vi "EverythingMultiFPGATest.vi"() -> ()   [LabVIEW 2017]
uses:
  Version Token.ctl
  Analog Replay/Settings.ctl
  Analog Replay/Input.ctl
  Analog Replay/Load Input.ctl
  Digital Pattern Generation/Load Input.ctl
  Digital Pattern Generation/Settings.ctl
  Digital Pattern Generation/Input.ctl
  ECU Event/Timing/Measure Output.ctl
  ECU Event/Timing/Measure Settings.ctl
  ECU Event/Timing/Capture Output.ctl
  Knock Sensor/Generate Input.ctl
  Knock Sensor/Cylinder Input.ctl
  Knock Sensor/Cylinder Settings.ctl
  Knock Sensor/Generate Settings.ctl
  Directional Speed/Load Input.ctl
  Directional Speed/Settings.ctl
  Directional Speed/Input.ctl
  APU/Settings.ctl
  APU/Input.ctl
  APU/Output.ctl
  APU/Shared Settings.ctl
  <vilib>/Platform/TimedLoop/XDataNode/timing_clust.ctl
  <vilib>/Platform/TimedLoop/XDataNode/nitl_modes.ctl
  <vilib>/Platform/TimedLoop/XDataNode/wakeup.ctl
  ECU Event/Timing/Capture Settings.ctl
  <vilib>/rvi/Emulation/niFpgaGetClockAttributes.vi
  <vilib>/rvi/Emulation/niFpgaSctlEmulationGetInTimedLoop.vi
  <vilib>/rvi/Emulation/niFpgaEmulationReportErrorSimple.vi
  <vilib>/rvi/DataTransferAndStorage/Container/Common/niFpgaContainerGetUniqueNameForEmu.vi
  <vilib>/rvi/DataTransferAndStorage/Container/Common/niFpgaContainerSetEmuInfo.vi
  <vilib>/rvi/eio/common/nirviEmuReportErrorAndStop.vi
  <vilib>/rvi/Emulation/niFpgaCriticalErrorInLSC.vi
  <vilib>/rvi/eio/common/nirviEmuTemplateMethod_errors.vi
  ECU Event/Timing/Measure Events (40MHz).vi
  <vilib>/rvi/DataTransferAndStorage/Container/Common/niFpgaContainerExecOnDevCompGetState.vi
  <vilib>/rvi/Emulation/niFpgaEmulationIsFPGAContextNoSignature.vi
  <vilib>/rvi/Memory/Memory_Emulation/niFpgaMemoryEmulationCacheClearOnFirstRun.vi
  <vilib>/rvi/Memory/Memory_Emulation/nirvimemoryEmulationManagerCache_MakeExclusive.vi
  <vilib>/rvi/Memory/Memory_Emulation/niFpgaMemoryEmulationValidateCache.vi
  <vilib>/rvi/Memory/Memory_Emulation/nirvimemoryEmulationManagerCache_InsertValue.vi
  <vilib>/Utility/error.llb/Clear Errors.vi
  <vilib>/rvi/Memory/Memory_Emulation/nirvimemoryEmulationManagerCache_ReleaseExclusive.vi
  <vilib>/rvi/Memory/Memory_Emulation/nirvimemoryEmulationManagerCache_GetValue.vi
  <vilib>/rvi/Memory/Memory_Emulation/nirvimemoryEmulationManagerCache_SetValue.vi
  <vilib>/rvi/Emulation/niFpgaProcessEmulError.vi
  <vilib>/rvi/LocalResourceManager/LocalResourceManager.xnode
  <vilib>/Platform/TimedLoop/XDataNode/XDataNode.xnode
  <vilib>/eio/EIONode/EIONode.xnode
  <vilib>/rvi/DataTransferAndStorage/Container/XNode/niFpgaContainer.xnode
  <vilib>/rvi/DataTransferAndStorage/Register/Emulation/niFpgaRegisterEmulationRefIn.vi
  <vilib>/Platform/TimedLoop/XDataNode/XDNodeRunTimeDep.lvlib
  Analog Replay/Analog Replay.lvlib
  Digital Pattern Generation/Digital Pattern Generation.lvlib
  ECU Event/Timing/ECU Event Timing.lvlib
  Knock Sensor/Knock Sensor.lvlib
  Directional Speed/Directional Speed.lvlib
  APU/APU.lvlib
  Engine Simulation Toolkit.lvlib
panel:
  in  "trigger line.apu 1":refnum<k21>="PXI_Trig0"
  in  "send trigger.apu 1":bool
  in  "shared settings.apu 1":T1 {"start" format="%#.15g"}
  in  "go.apu 1":bool
  in  "master.apu 1":bool
  out "output.apu 1":T2 caption="output"
  in  "input.apu 1":T3={"desired speed"=0.0, "reset"=TRUE} caption="input"
  in  "settings.apu 1":T4 caption="settings"
  out "Digital Pattern Test.apu 1":T5
  in  "load input.Dir Speed DIO0":T6
  in  "input.Dir Speed DIO0":T7
  in  "settings.Dir Speed DIO0":T8
  in  "input.Dir Speed DIO1":T7
  in  "settings.Dir Speed DIO1":T8
  in  "load input.Dir Speed DIO1":T6
  in  "settings.Knock AO 3":T9
  in  "settings.Knock AO 3.Cylinder 1":T10
  in  "settings.Knock AO 3.Cylinder 2":T10
  in  "settings.Knock AO 3.Cylinder 3":T10
  in  "settings.Knock AO 3.Cylinder 4":T10
  in  "input.Knock AO 3.Cylinder 1":T11
  in  "input.Knock AO 3.Cylinder 2":T11
  in  "input.Knock AO 3.Cylinder 3":T11
  in  "input.Knock AO 3.Cylinder 4":T11
  in  "input.Knock AO 3":T12
  in  "settings.Knock AO 3.Cylinder 5":T10
  in  "settings.Knock AO 3.Cylinder 6":T10
  in  "input.Knock AO 3.Cylinder 5":T11
  in  "input.Knock AO 3.Cylinder 6":T11
  in  "settings.Knock AO 2.Cylinder 5":T10
  in  "settings.Knock AO 2.Cylinder 6":T10
  in  "input.Knock AO 2.Cylinder 5":T11={"probability compare"=65535, "high freq scaler"=0.0, "trigger position"=0}
  in  "input.Knock AO 2.Cylinder 6":T11={"probability compare"=65535, "high freq scaler"=0.0, "trigger position"=0}
  in  "settings.Knock AO 2":T9
  in  "settings.Knock AO 2.Cylinder 1":T10
  in  "settings.Knock AO 2.Cylinder 2":T10
  in  "settings.Knock AO 2.Cylinder 3":T10
  in  "settings.Knock AO 2.Cylinder 4":T10
  in  "input.Knock AO 2.Cylinder 1":T11={"probability compare"=65535, "high freq scaler"=0.0, "trigger position"=0}
  in  "input.Knock AO 2.Cylinder 2":T11={"probability compare"=65535, "high freq scaler"=0.0, "trigger position"=0}
  in  "input.Knock AO 2.Cylinder 3":T11={"probability compare"=65535, "high freq scaler"=0.0, "trigger position"=0}
  in  "input.Knock AO 2.Cylinder 4":T11={"probability compare"=65535, "high freq scaler"=0.0, "trigger position"=0}
  in  "input.Knock AO 2":T12
  out "capture.Multi Event DIO 15.Event 4":T13
  out "capture.Multi Event DIO 15.Event 3":T13
  out "capture.Multi Event DIO 15.Event 2":T13
  out "capture.Multi Event DIO 14.Event 4":T13
  out "capture.Multi Event DIO 14.Event 3":T13
  out "capture.Multi Event DIO 14.Event 2":T13
  out "capture.Multi Event DIO 13.Event 4":T13
  out "capture.Multi Event DIO 13.Event 3":T13
  out "capture.Multi Event DIO 13.Event 2":T13
  out "capture.Multi Event DIO 12.Event 4":T13
  out "capture.Multi Event DIO 12.Event 3":T13
  out "capture.Multi Event DIO 12.Event 2":T13
  out "capture.Multi Event DIO 11.Event 4":T13
  out "capture.Multi Event DIO 11.Event 3":T13
  out "capture.Multi Event DIO 11.Event 2":T13
  out "capture.Multi Event DIO 10.Event 4":T13
  out "capture.Multi Event DIO 10.Event 3":T13
  out "capture.Multi Event DIO 10.Event 2":T13
  out "capture.Multi Event DIO 10.Event 1":T13
  out "capture.Multi Event DIO 11.Event 1":T13
  out "capture.Multi Event DIO 12.Event 1":T13
  out "capture.Multi Event DIO 13.Event 1":T13
  out "capture.Multi Event DIO 14.Event 1":T13
  out "capture.Multi Event DIO 15.Event 1":T13
  in  "settings.Multi Event DIO 10":T14
  in  "settings.Multi Event DIO 11":T14
  in  "settings.Multi Event DIO 12":T14
  in  "settings.Multi Event DIO 13":T14
  in  "settings.Multi Event DIO 14":T14
  in  "settings.Multi Event DIO 15":T14
  out "status.Multi Event DIO 10":T15
  out "status.Multi Event DIO 11":T15
  out "status.Multi Event DIO 12":T15
  out "status.Multi Event DIO 13":T15
  out "status.Multi Event DIO 14":T15
  out "status.Multi Event DIO 15":T15
  out "capture.Event DIO 4.Event 1":T13
  out "capture.Event DIO 5.Event 1":T13
  out "capture.Event DIO 6.Event 1":T13
  out "capture.Event DIO 7.Event 1":T13
  out "capture.Event DIO 8.Event 1":T13
  out "capture.Event DIO 9.Event 1":T13
  in  "settings.Event DIO 4":T14
  in  "settings.Event DIO 5":T14
  in  "settings.Event DIO 6":T14
  in  "settings.Event DIO 7":T14
  in  "settings.Event DIO 8":T14
  in  "settings.Event DIO 9":T14
  out "status.Event DIO 4":T15
  out "status.Event DIO 5":T15
  out "status.Event DIO 6":T15
  out "status.Event DIO 7":T15
  out "status.Event DIO 8":T15
  out "status.Event DIO 9":T15
  in  "load input.Pattern DIO 3":T16
  in  "load input.Pattern DIO 2":T16
  in  "load input.Pattern DIO 1":T16
  in  "input.Pattern DIO 0":T17
  in  "settings.Pattern DIO 0":T18
  in  "input.Pattern DIO 1":T17
  in  "settings.Pattern DIO 1":T18
  in  "input.Pattern DIO 2":T17
  in  "settings.Pattern DIO 2":T18
  in  "input.Pattern DIO 3":T17
  in  "settings.Pattern DIO 3":T18
  in  "load input.Pattern DIO 0":T16
  in  "load input.replay AO 1":T19={"Data"=[0, 0, 0, 0, 0, 0, 0, 0, 0, 0, 0, 0, 0, 0, 0, 0], "LoadOffset"=0, "Done"=FALSE} caption="input"
  in  "load input.replay AO 0":T19={"Data"=[0, 0, 0, 0, 0, 0, 0, 0, 0, 0, 0, 0, 0, 0, 0, 0], "LoadOffset"=0, "Done"=FALSE} caption="input"
  in  "input.replay AO 0":T20 caption="input"
  in  "input.replay AO 1":T20 caption="input"
  in  "settings.replay AO 1":T21 caption="settings"
  in  "settings.replay AO 0":T21 caption="settings"
  in  "est.version":T22
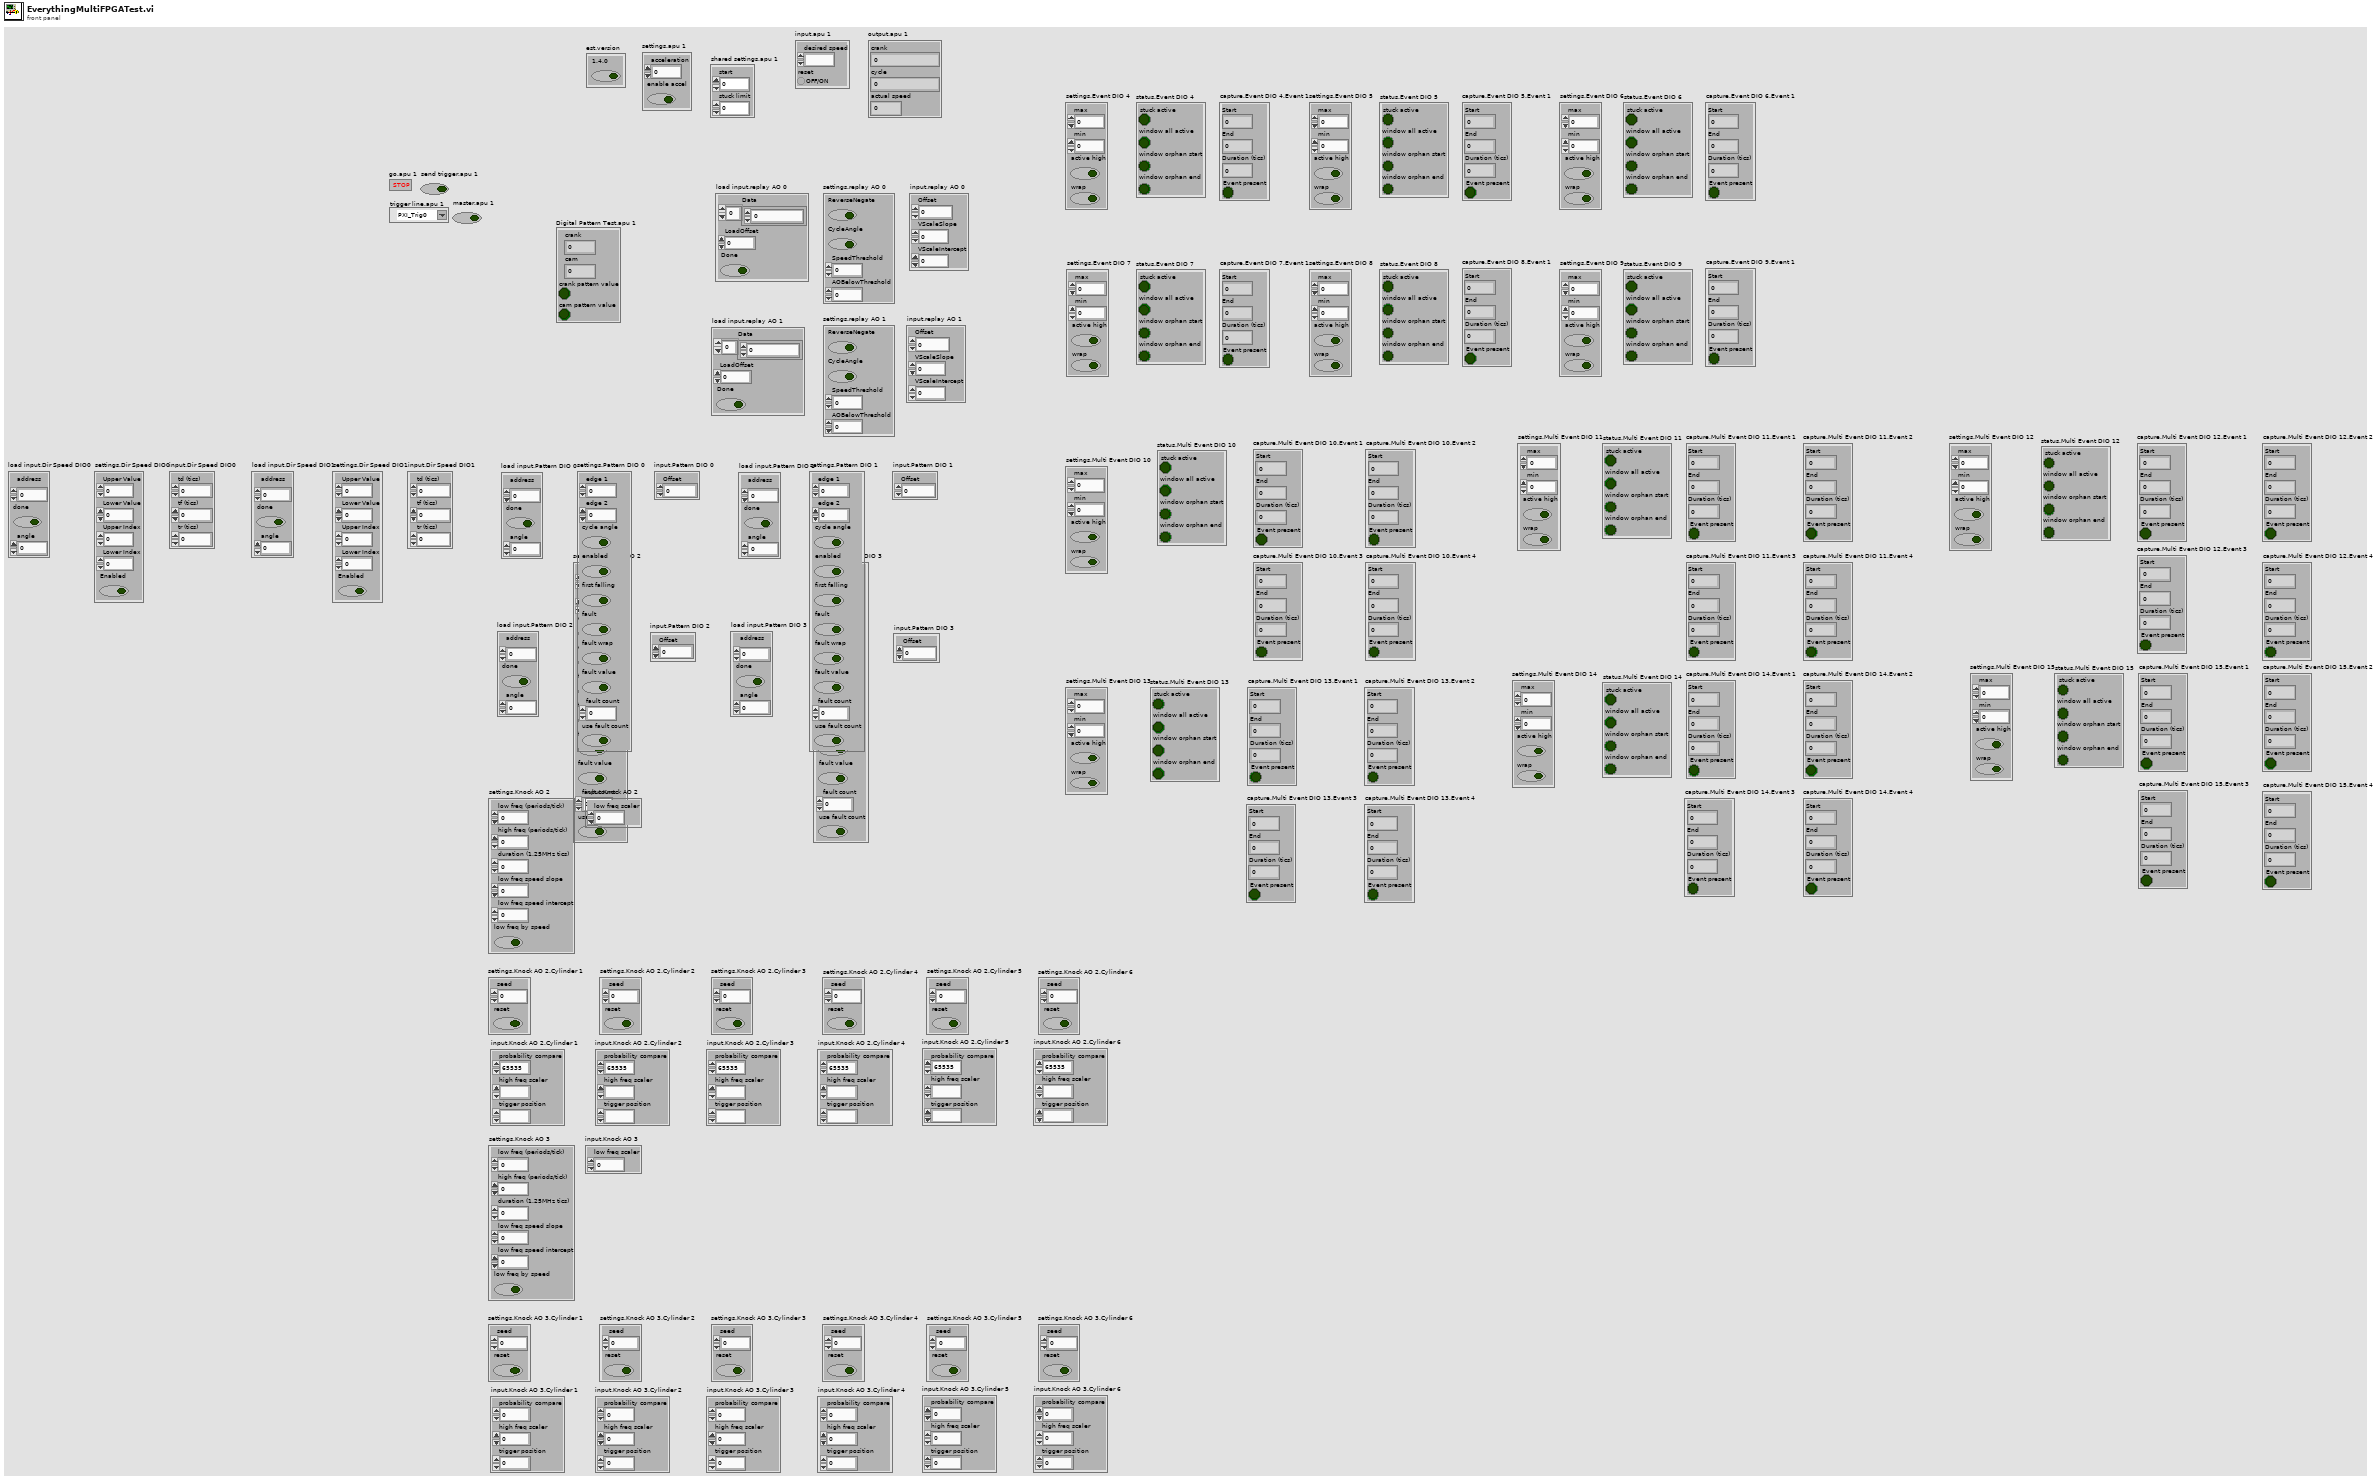
[diagram p1: front panel]
types:
  T1 = typedef "Engine Simulation Toolkit.lvlib/APU.lvlib/Shared Settings.ctl" = cluster{"start":fxp<+,17,17>, "stuck limit":fxp<+,18,18>}
  T2 = typedef "Engine Simulation Toolkit.lvlib/APU.lvlib/Output.ctl" = cluster{"crank":u16, "cycle":u16, "actual speed":fxp<+/-,23,2>}
  T3 = typedef "Engine Simulation Toolkit.lvlib/APU.lvlib/Input.ctl" = cluster{"desired speed":fxp<+/-,23,2>, "reset":bool}
  T4 = typedef "Engine Simulation Toolkit.lvlib/APU.lvlib/Settings.ctl" = cluster{"acceleration":fxp<+,18,-20>, "enable accel":bool}
  T5 = cluster{"crank":u16, "cam":u16, "crank pattern value":bool, "cam pattern value":bool}
  T6 = typedef "Engine Simulation Toolkit.lvlib/Directional Speed.lvlib/Load Input.ctl" = cluster{"address":fxp<+,10,10>, "done":bool, "angle":u16}
  T7 = typedef "Engine Simulation Toolkit.lvlib/Directional Speed.lvlib/Input.ctl" = cluster{"td (tics)":u16, "tf (tics)":u16, "tr (tics)":u16}
  T8 = typedef "Engine Simulation Toolkit.lvlib/Directional Speed.lvlib/Settings.ctl" = cluster{"Upper Value":u16, "Lower Value":u16, "Upper Index":fxp<+,10,10>, "Lower Index":fxp<+,10,10>, "Enabled":bool}
  T9 = typedef "Engine Simulation Toolkit.lvlib/Knock Sensor.lvlib/Generate Settings.ctl" = cluster{"low freq (periods/tick)":fxp<+,32,0>, "high freq (periods/tick)":fxp<+,32,0>, "duration (1.25MHz tics)":fxp<+,18,18>, "low freq speed slope":fxp<+,16,-3>, "low freq speed intercept":fxp<+,10,-10>, "low freq by speed":bool}
  T10 = typedef "Engine Simulation Toolkit.lvlib/Knock Sensor.lvlib/Cylinder Settings.ctl" = cluster{"seed":u16, "reset":bool}
  T11 = typedef "Engine Simulation Toolkit.lvlib/Knock Sensor.lvlib/Cylinder Input.ctl" = cluster{"probability compare":u16, "high freq scaler":fxp<+,10,0>, "trigger position":u16}
  T12 = typedef "Engine Simulation Toolkit.lvlib/Knock Sensor.lvlib/Generate Input.ctl" = cluster{"low freq scaler":fxp<+,10,0>}
  T13 = typedef "Engine Simulation Toolkit.lvlib/ECU Event Timing.lvlib/Capture Output.ctl" = cluster{"Start":u16, "End":u16, "Duration (tics)":fxp<+,18,18>, "Event present":bool}
  T14 = typedef "Engine Simulation Toolkit.lvlib/ECU Event Timing.lvlib/Measure Settings.ctl" = cluster{"max":u16, "min":u16, "active high":bool, "wrap":bool}
  T15 = typedef "Engine Simulation Toolkit.lvlib/ECU Event Timing.lvlib/Measure Output.ctl" = cluster{"stuck active":bool, "window all active":bool, "window orphan start":bool, "window orphan end":bool}
  T16 = typedef "Engine Simulation Toolkit.lvlib/Digital Pattern Generation.lvlib/Load Input.ctl" = cluster{"address":fxp<+,11,11>, "done":bool, "angle":u16}
  T17 = typedef "Engine Simulation Toolkit.lvlib/Digital Pattern Generation.lvlib/Input.ctl" = cluster{"Offset":i16}
  T18 = typedef "Engine Simulation Toolkit.lvlib/Digital Pattern Generation.lvlib/Settings.ctl" = cluster{"edge 1":u16, "edge 2":u16, "cycle angle":bool, "enabled":bool, "first falling":bool, "fault":bool, "fault wrap":bool, "fault value":bool, "fault count":fxp<+,4,4>, "use fault count":bool}
  T19 = typedef "Engine Simulation Toolkit.lvlib/Analog Replay.lvlib/Load Input.ctl" = cluster{"Data":i16[], "LoadOffset":u16, "Done":bool}
  T20 = typedef "Engine Simulation Toolkit.lvlib/Analog Replay.lvlib/Input.ctl" = cluster{"Offset":i16, "VScaleSlope":fxp<+,18,6>, "VScaleIntercept":fxp<+/-,18,3>}
  T21 = typedef "Engine Simulation Toolkit.lvlib/Analog Replay.lvlib/Settings.ctl" = cluster{"ReverseNegate":bool, "CycleAngle":bool, "SpeedThreshold":fxp<+/-,23,2>, "AOBelowThreshold":i16}
  T22 = typedef "Engine Simulation Toolkit.lvlib/Version Token.ctl" = cluster{"1.4.0":bool}
  T23 = typedef "XDNodeRunTimeDep.lvlib/timing_clust.ctl" = cluster{"Expected End [f-1]":u64, "Actual End [f-1]":u64, "Finished Late? [f-1]":bool, "Expected End [i-1]":u64, "Actual End [i-1]":u64, "Finished Late? [i-1]":bool, "Expected Start [i]":u64, "Actual Start [i]":u64, "Expected Start [f]":u64, "Actual Start [f]":u64, "Source Name":string, "Structure Name":string, "Period":i64, "Deadline":i64, "Offset":i64, "Start":i64, "Priority":i32, "Timeout":i32, "Mode":T24, "Wakeup Reason":T25, "Error":errorcluster, "Source Type":string, "Secondary Source Type":string, "Global End Time":u64, "Global Start Time":u64, "Frame Duration":u64, "Iteration Duration":u64, "Assigned CPU":i32, "I/O Scan Engine Mode":u32}
  T24 = typedef "XDNodeRunTimeDep.lvlib/nitl_modes.ctl" = enum32{"No Change", "Process missed periods, maintain original phase", "Discard missed periods, maintain original phase", "Process missed periods, ignore original phase", "Discard missed periods, ignore original phase"}
  T25 = typedef "XDNodeRunTimeDep.lvlib/wakeup.ctl" = enum32{"Normal", "Aborted", "Asynchronous wakeup", "Timing source error", "Timed loop error", "Timeout"}
  T26 = typedef "Engine Simulation Toolkit.lvlib/Directional Speed.lvlib/Load Data.ctl" = cluster{"max address":fxp<+,10,10>, "Memory":refnum<k21>}
  T27 = typedef "Engine Simulation Toolkit.lvlib/APU.lvlib/Register Bus.ctl" = cluster{"Speed":refnum<k21>, "Crank Angle":refnum<k21>, "Cycle Angle":refnum<k21>, "Crank Count":refnum<k21>, "Cycle Count":refnum<k21>, "1.25 MHz Counter":refnum<k21>, "Crank Rollover":refnum<k21>, "Cycle Rollover":refnum<k21>, "shared settings":T1}
  T28 = typedef "Engine Simulation Toolkit.lvlib/Digital Pattern Generation.lvlib/Load Data.ctl" = cluster{"max address":fxp<+,11,11>, "memory":refnum<k21>}
  T29 = typedef "Engine Simulation Toolkit.lvlib/Knock Sensor.lvlib/Triggered Cylinder Data.ctl" = cluster{"trigger knock":bool, "high freq scaler":fxp<+,10,0>}
  T30 = typedef "Engine Simulation Toolkit.lvlib/ECU Event Timing.lvlib/Capture Settings.ctl" = u8
  T31 = typedef "Engine Simulation Toolkit.lvlib/ECU Event Timing.lvlib/Measured Data.ctl" = cluster{"start":u16, "end":u16, "duration (tics)":fxp<+,18,18>, "window end":bool, "window begin":bool, "pulse end":bool, "pulse #":u8}
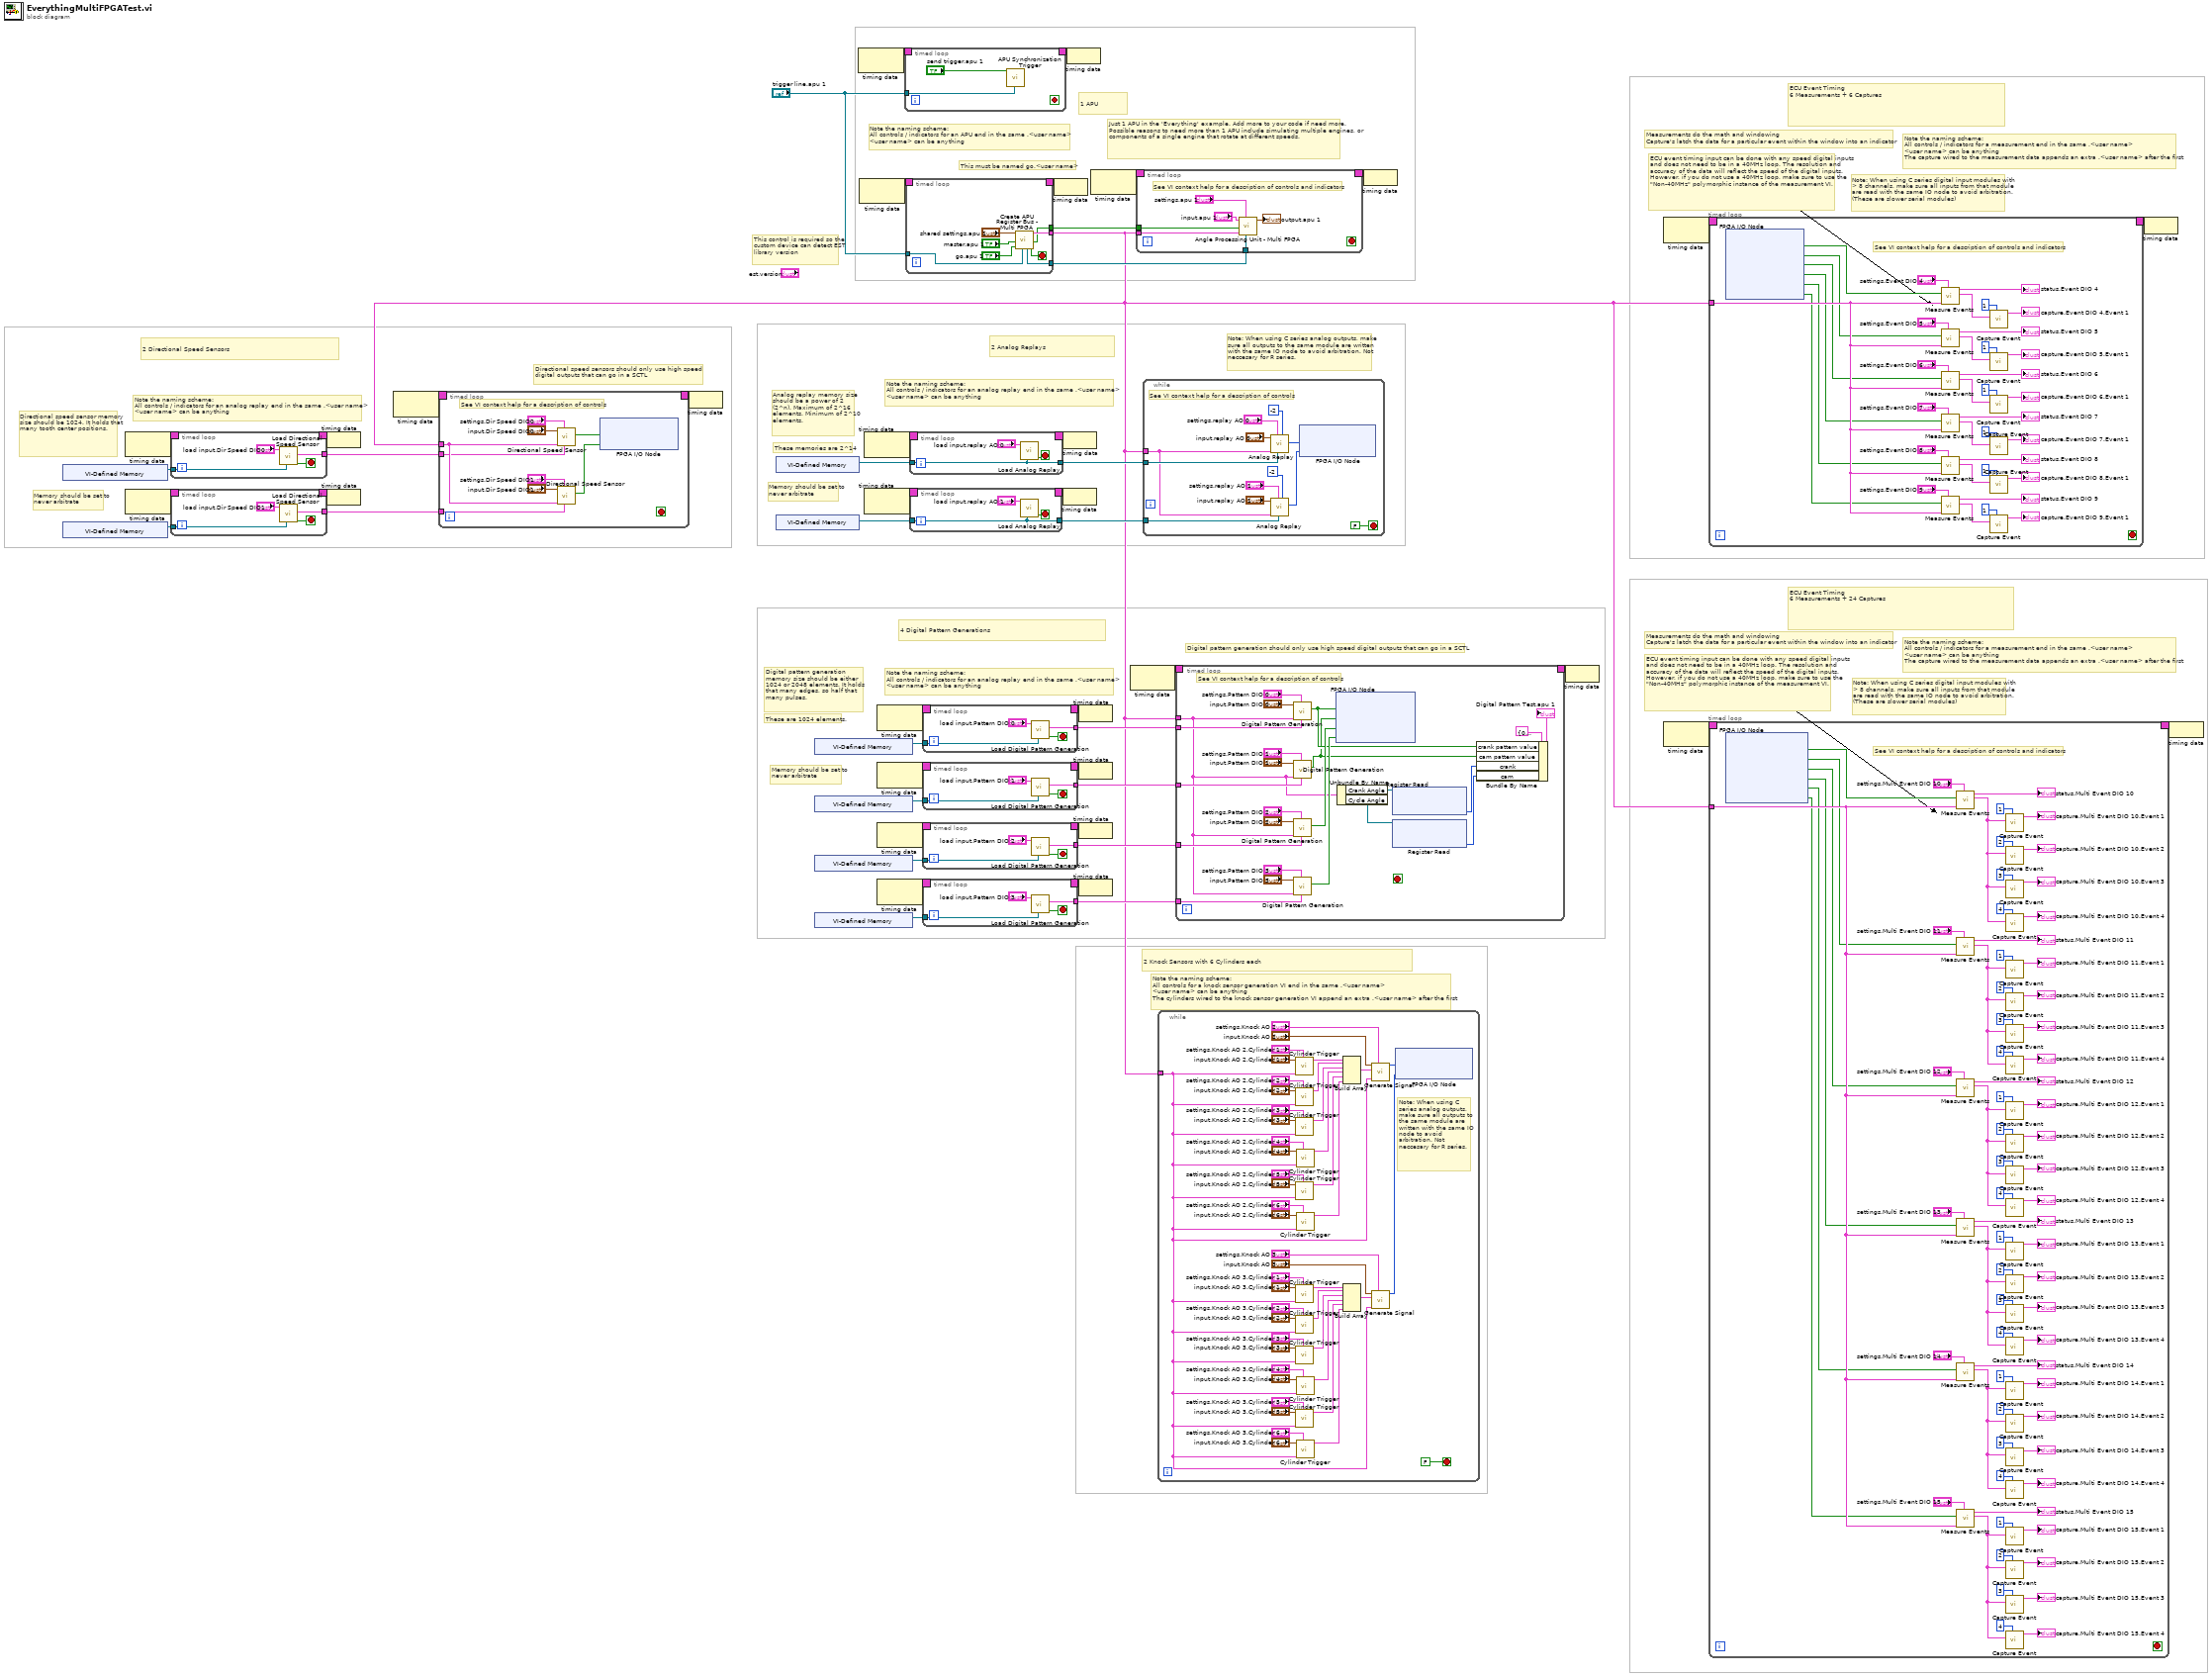
[diagram p0: block diagram]
diagram:
  # "This must be named go.<user name>"
  # "1 APU"
  # "Note the naming scheme: \nAll controls / indicators for an APU end in the same .<user name>\n<user name> can be anything"
  # "Just 1 APU in the 'Everything' example. Add more to your code if need more. Possible reasons to need more than 1 APU include simulating multiple engines, or components of a single engine that rotate at different speeds."
  # "ECU event timing input can be done with any speed digital inputs and does not need to be in a 40MHz loop. The resolution and accuracy of the data will reflect the speed of the digital inputs. However, if you do not use a 40MHz loop, make sure to use the \"Non-40MHz\" polymorphic instance of the measurement VI."
  # "Memory should be set to never arbitrate"
  # "Memory should be set to never arbitrate"
  # "Memory should be set to never arbitrate"
  # "Note the naming scheme: \nAll controls / indicators for an analog replay end in the same .<user name>\n<user name> can be anything"
  # "Directional speed sensor memory size should be 1024. It holds that many tooth center positions."
  # "Directional speed sensors should only use high speed digital outputs that can go in a SCTL"
  # "2 Directional Speed Sensors"
  # "Note the naming scheme: \nAll controls for a knock sensor generation VI end in the same .<user name>\n<user name> can be anything\nThe cylinders wired to the knock sensor generation VI append an extra .<user name> after the first"
  # "2 Knock Sensors with 6 Cylinders each"
  # "Note: When using C series digital input modules with > 8 channels, make sure all inputs from that module are read with the same IO node to avoid arbitration. (These are slower serial modules)"
  # "Measurements do the math and windowing\nCapture's latch the data for a particular event within the window into an indicator"
  # "ECU Event Timing\n6 Measurements + 24 Captures"
  # "Note the naming scheme: \nAll controls / indicators for a measurement end in the same .<user name>\n<user name> can be anything\nThe capture wired to the measurement data appends an extra .<user name> after the first"
  # "Note: When using C series digital input modules with > 8 channels, make sure all inputs from that module are read with the same IO node to avoid arbitration. (These are slower serial modules)"
  # "Measurements do the math and windowing\nCapture's latch the data for a particular event within the window into an indicator"
  # "ECU Event Timing\n6 Measurements + 6 Captures"
  # "Note the naming scheme: \nAll controls / indicators for a measurement end in the same .<user name>\n<user name> can be anything\nThe capture wired to the measurement data appends an extra .<user name> after the first"
  # "ECU event timing input can be done with any speed digital inputs and does not need to be in a 40MHz loop. The resolution and accuracy of the data will reflect the speed of the digital inputs. However, if you do not use a 40MHz loop, make sure to use the \"Non-40MHz\" polymorphic instance of the measurement VI."
  # "Digital pattern generation should only use high speed digital outputs that can go in a SCTL"
  # "4 Digital Pattern Generations"
  # "Note the naming scheme: \nAll controls / indicators for an analog replay end in the same .<user name>\n<user name> can be anything"
  # "These are 1024 elements."
  # "Digital pattern generation memory size should be either 1024 or 2048 elements. It holds that many edges, so half that many pulses."
  # "Note: When using C series analog outputs, make sure all outputs to the same module are written with the same IO node to avoid arbitration. Not neccesary for R series."
  # "2 Analog Replays"
  # "These memories are 2^14"
  # "Note the naming scheme: \nAll controls / indicators for an analog replay end in the same .<user name>\n<user name> can be anything"
  # "Analog replay memory size should be a power of 2 (2^n). Maximum of 2^16 elements. Minimum of 2^10 elements."
  # "This control is required so the custom device can detect EST library version"
  n1 = xnode "VI-Defined Memory"() -> ("Memory Out"=w11:refnum<k21>)
  n2 = xnode "VI-Defined Memory"() -> ("Memory Out"=w13:refnum<k21>)
  n3 = node-c288() -> (w20:T23)  [unwired: 1 in]
  n4 = node-c288() -> (w16:T23)  [unwired: 1 in]
  n5 = timed-loop {
    timing: w20 -> [_]
    timing-out: [_] -> w19
    tunnel: w11 -> [w53]
    tunnel: [w52] -> w12
    stop <- w54 stop-if-true
    n6 = call "Load Directional Speed Sensor.vi"("Memory In"=w53, "load input.<user name>"="load input.Dir Speed DIO0") -> ("done"=w54:bool, "load data"=w52:T26)  [unwired: 8 in]
  }
  n7 = timed-loop {
    timing: w16 -> [_]
    timing-out: [_] -> w15
    tunnel: w13 -> [w59]
    tunnel: [w58] -> w14
    stop <- w60 stop-if-true
    n8 = call "Load Directional Speed Sensor.vi"("Memory In"=w59, "load input.<user name>"="load input.Dir Speed DIO1") -> ("done"=w60:bool, "load data"=w58:T26)  [unwired: 8 in]
  }
  n9 = node-c288(w19) -> ()
  n10 = node-c288(w15) -> ()
  n11 = node-c288() -> (w18:T23)  [unwired: 1 in]
  n12 = xnode "VI-Defined Memory"() -> ("Memory Out"=w45:refnum<k21>)
  n13 = xnode "VI-Defined Memory"() -> ("Memory Out"=w46:refnum<k21>)
  n14 = xnode "VI-Defined Memory"() -> ("Memory Out"=w38:refnum<k21>)
  n15 = xnode "VI-Defined Memory"() -> ("Memory Out"=w34:refnum<k21>)
  n16 = xnode "VI-Defined Memory"() -> ("Memory Out"=w31:refnum<k21>)
  n17 = xnode "VI-Defined Memory"() -> ("Memory Out"=w28:refnum<k21>)
  n18 = node-c288() -> (w6:T23)  [unwired: 1 in]
  n19 = node-c288() -> (w8:T23)  [unwired: 1 in]
  n20 = node-c288() -> (w50:T23)  [unwired: 1 in]
  n21 = node-c288() -> (w48:T23)  [unwired: 1 in]
  n22 = node-c288() -> (w42:T23)  [unwired: 1 in]
  n23 = node-c288() -> (w36:T23)  [unwired: 1 in]
  n24 = node-c288() -> (w33:T23)  [unwired: 1 in]
  n25 = node-c288() -> (w30:T23)  [unwired: 1 in]
  n26 = timed-loop {
    timing: w6 -> [_]
    timing-out: [_] -> w5
    tunnel: "trigger line.apu 1" -> [w63]
    stop <- _ stop-if-true
    n27 = call "APU Synchronization Trigger.vi"("trigger line.<user name>"=w63, "send trigger.<user name>"="send trigger.apu 1") -> ()  [unwired: 10 in]
  }
  n28 = timed-loop {
    timing: w8 -> [_]
    timing-out: [_] -> w7
    tunnel: [w73] -> w1
    tunnel: [w70] -> w4
    tunnel: [w69] -> w3
    tunnel: "trigger line.apu 1" -> [w67]
    stop <- w68 stop-if-true
    n29 = call "Create APU Register Bus - Multi FPGA.vi"("trigger line.<user name>"=w67, "go.<user name>"="go.apu 1", "master.<user name>"="master.apu 1", "shared settings.<user name>"="shared settings.apu 1") -> ("go?"=w68:bool, "master?"=w69:bool, "register bus"=w73:T27, "trigger line"=w70:refnum<k21>)  [unwired: 4 in]
  }
  n30 = timed-loop {
    tunnel: w1 -> [w79]
    timing: w18 -> [_]
    timing-out: [_] -> w17
    tunnel: w12 -> [w78]
    tunnel: w14 -> [w77]
    stop <- _ stop-if-true
    # "See VI context help for a description of controls"
    n31 = call "Directional Speed Sensor.vi"("load data"=w78, "settings.<user name>"="settings.Dir Speed DIO0", "register bus"=w79, "input.<user name>"="input.Dir Speed DIO0") -> ("digial output"=w82:bool)  [unwired: 7 in]
    n32 = call "Directional Speed Sensor.vi"("load data"=w77, "settings.<user name>"="settings.Dir Speed DIO1", "register bus"=w79, "input.<user name>"="input.Dir Speed DIO1") -> ("digial output"=w83:bool)  [unwired: 7 in]
    n33 = xnode "FPGA I/O Node"("Connector1/DIO0"=w82, "Connector1/DIO1"=w83) -> ()  [unwired: 2 in, 2 out]
  }
  n34 = node-c288(w17) -> ()
  n35 = timed-loop {
    timing: w50 -> [_]
    timing-out: [_] -> w49
    tunnel: w45 -> [w88]
    tunnel: [w88] -> w44
    stop <- w89 stop-if-true
    n36 = call "Load Analog Replay.vi"("memory"=w88, "load input.<user name>"="load input.replay AO 0") -> ("done"=w89:bool)  [unwired: 9 in]
  }
  n37 = timed-loop {
    timing: w48 -> [_]
    timing-out: [_] -> w47
    tunnel: w46 -> [w93]
    tunnel: [w93] -> w43
    stop <- w94 stop-if-true
    n38 = call "Load Analog Replay.vi"("memory"=w93, "load input.<user name>"="load input.replay AO 1") -> ("done"=w94:bool)  [unwired: 9 in]
  }
  n39 = timed-loop {
    timing: w42 -> [_]
    timing-out: [_] -> w41
    tunnel: w38 -> [w100]
    tunnel: [w99] -> w37
    stop <- w101 stop-if-true
    n40 = call "Load Digital Pattern Generation.vi"("memory"=w100, "load input.<user name>"="load input.Pattern DIO 0") -> ("done"=w101:bool, "load data"=w99:T28)  [unwired: 8 in]
  }
  n41 = timed-loop {
    timing: w36 -> [_]
    timing-out: [_] -> w35
    tunnel: w34 -> [w106]
    tunnel: [w105] -> w25
    stop <- w107 stop-if-true
    n42 = call "Load Digital Pattern Generation.vi"("memory"=w106, "load input.<user name>"="load input.Pattern DIO 1") -> ("done"=w107:bool, "load data"=w105:T28)  [unwired: 8 in]
  }
  n43 = timed-loop {
    timing: w33 -> [_]
    timing-out: [_] -> w32
    tunnel: w31 -> [w112]
    tunnel: [w111] -> w26
    stop <- w113 stop-if-true
    n44 = call "Load Digital Pattern Generation.vi"("memory"=w112, "load input.<user name>"="load input.Pattern DIO 2") -> ("done"=w113:bool, "load data"=w111:T28)  [unwired: 8 in]
  }
  n45 = timed-loop {
    timing: w30 -> [_]
    timing-out: [_] -> w29
    tunnel: w28 -> [w118]
    tunnel: [w117] -> w27
    stop <- w119 stop-if-true
    n46 = call "Load Digital Pattern Generation.vi"("memory"=w118, "load input.<user name>"="load input.Pattern DIO 3") -> ("done"=w119:bool, "load data"=w117:T28)  [unwired: 8 in]
  }
  n47 = node-c288(w7) -> ()
  n48 = node-c288(w47) -> ()
  n49 = node-c288(w49) -> ()
  n50 = node-c288(w5) -> ()
  n51 = node-c288(w41) -> ()
  n52 = node-c288(w35) -> ()
  n53 = node-c288(w32) -> ()
  n54 = node-c288(w29) -> ()
  n55 = node-c288() -> (w10:T23)  [unwired: 1 in]
  n56 = node-c288() -> (w40:T23)  [unwired: 1 in]
  n57 = timed-loop {
    timing: w10 -> [_]
    timing-out: [_] -> w9
    tunnel: w1 -> [w124]
    tunnel: w4 -> [w123]
    tunnel: w3 -> [w122]
    stop <- _ stop-if-true
    # "See VI context help for a description of controls and indicators"
    n58 = call "Angle Processing Unit - Multi FPGA.vi"("trigger line.<user name>"=w123, "settings.<user name>"="settings.apu 1", "register bus"=w124, "master"=w122, "input.<user name>"="input.apu 1") -> ("output.<user name>"=→"output.apu 1":T2)  [unwired: 6 in]
  }
  n59 = while {
    tunnel: w44 -> [w141]
    tunnel: w1 -> [w130]
    tunnel: w43 -> [w138]
    stop <- FALSE stop-if-true
    # "See VI context help for a description of controls"
    n60 = call "Analog Replay.vi"("shift"=i8 -2, "memory"=w141, "settings.<user name>"="settings.replay AO 0", "register bus"=w130, "input.<user name>"="input.replay AO 0") -> ("analog value"=w134:i16)  [unwired: 6 in]
    n61 = call "Analog Replay.vi"("shift"=i8 -2, "memory"=w138, "settings.<user name>"="settings.replay AO 1", "register bus"=w130, "input.<user name>"="input.replay AO 1") -> ("analog value"=w133:i16)  [unwired: 6 in]
    n62 = xnode "FPGA I/O Node"("Connector0/AO0"=w134, "Connector0/AO1"=w133) -> ()  [unwired: 2 in, 2 out]
  }
  n63 = while {
    tunnel: w1 -> [w143]
    stop <- FALSE stop-if-true
    # "Note: When using C series analog outputs, make sure all outputs to the same module are written with the same IO node to avoid arbitration. Not neccesary for R series."
    n64 = call "Cylinder Trigger.vi"("settings.<user name>"="settings.Knock AO 2.Cylinder 1", "register bus"=w143, "input.<user name>"="input.Knock AO 2.Cylinder 1") -> ("triggered knock data"=w187:T29)  [unwired: 8 in]
    n65 = call "Cylinder Trigger.vi"("settings.<user name>"="settings.Knock AO 2.Cylinder 2", "register bus"=w143, "input.<user name>"="input.Knock AO 2.Cylinder 2") -> ("triggered knock data"=w186:T29)  [unwired: 8 in]
    n66 = call "Cylinder Trigger.vi"("settings.<user name>"="settings.Knock AO 2.Cylinder 3", "register bus"=w143, "input.<user name>"="input.Knock AO 2.Cylinder 3") -> ("triggered knock data"=w185:T29)  [unwired: 8 in]
    n67 = call "Cylinder Trigger.vi"("settings.<user name>"="settings.Knock AO 2.Cylinder 5", "register bus"=w143, "input.<user name>"="input.Knock AO 2.Cylinder 5") -> ("triggered knock data"=w166:T29)  [unwired: 8 in]
    n68 = call "Cylinder Trigger.vi"("settings.<user name>"="settings.Knock AO 3.Cylinder 1", "register bus"=w143, "input.<user name>"="input.Knock AO 3.Cylinder 1") -> ("triggered knock data"=w144:T29)  [unwired: 8 in]
    n69 = call "Cylinder Trigger.vi"("settings.<user name>"="settings.Knock AO 3.Cylinder 2", "register bus"=w143, "input.<user name>"="input.Knock AO 3.Cylinder 2") -> ("triggered knock data"=w145:T29)  [unwired: 8 in]
    n70 = call "Cylinder Trigger.vi"("settings.<user name>"="settings.Knock AO 3.Cylinder 3", "register bus"=w143, "input.<user name>"="input.Knock AO 3.Cylinder 3") -> ("triggered knock data"=w146:T29)  [unwired: 8 in]
    n71 = call "Cylinder Trigger.vi"("settings.<user name>"="settings.Knock AO 3.Cylinder 5", "register bus"=w143, "input.<user name>"="input.Knock AO 3.Cylinder 5") -> ("triggered knock data"=w163:T29)  [unwired: 8 in]
    n72 = call "Cylinder Trigger.vi"("settings.<user name>"="settings.Knock AO 2.Cylinder 4", "register bus"=w143, "input.<user name>"="input.Knock AO 2.Cylinder 4") -> ("triggered knock data"=w184:T29)  [unwired: 8 in]
    n73 = call "Cylinder Trigger.vi"("settings.<user name>"="settings.Knock AO 2.Cylinder 6", "register bus"=w143, "input.<user name>"="input.Knock AO 2.Cylinder 6") -> ("triggered knock data"=w165:T29)  [unwired: 8 in]
    n74 = call "Cylinder Trigger.vi"("settings.<user name>"="settings.Knock AO 3.Cylinder 4", "register bus"=w143, "input.<user name>"="input.Knock AO 3.Cylinder 4") -> ("triggered knock data"=w147:T29)  [unwired: 8 in]
    n75 = call "Cylinder Trigger.vi"("settings.<user name>"="settings.Knock AO 3.Cylinder 6", "register bus"=w143, "input.<user name>"="input.Knock AO 3.Cylinder 6") -> ("triggered knock data"=w164:T29)  [unwired: 8 in]
    n76 = Build Array(w187, w186, w185, w184, w166, w165) -> (w183:T29[])
    n77 = Build Array(w144, w145, w146, w147, w163, w164) -> (w148:T29[])
    n78 = call "Generate Signal.vi"("settings.<user name>"="settings.Knock AO 2", "register bus"=w143, "triggered knock data"=w183, "input.<user name>"="input.Knock AO 2") -> ("knock signal"=w171:i16)  [unwired: 7 in]
    n79 = call "Generate Signal.vi"("settings.<user name>"="settings.Knock AO 3", "register bus"=w143, "triggered knock data"=w148, "input.<user name>"="input.Knock AO 3") -> ("knock signal"=w142:i16)  [unwired: 7 in]
    n80 = xnode ("FPGA I/O Node")("Connector0/AO2"=w171, "Connector0/AO3"=w142) -> ()  [unwired: 2 in, 2 out]
  }
  n81 = timed-loop {
    tunnel: w1 -> [w193]
    timing: w40 -> [_]
    timing-out: [_] -> w39
    tunnel: w37 -> [w200]
    tunnel: w25 -> [w194]
    tunnel: w26 -> [w199]
    tunnel: w27 -> [w198]
    stop <- _ stop-if-true
    # "See VI context help for a description of controls"
    n82 = call "Digital Pattern Generation.vi"("load data"=w200, "settings.<user name>"="settings.Pattern DIO 0", "register bus"=w193, "input.<user name>"="input.Pattern DIO 0") -> ("digial output"=w196:bool)  [unwired: 7 in]
    n83 = call "Digital Pattern Generation.vi"("load data"=w194, "settings.<user name>"="settings.Pattern DIO 1", "register bus"=w193, "input.<user name>"="input.Pattern DIO 1") -> ("digial output"=w195:bool)  [unwired: 7 in]
    n84 = call "Digital Pattern Generation.vi"("load data"=w199, "settings.<user name>"="settings.Pattern DIO 2", "register bus"=w193, "input.<user name>"="input.Pattern DIO 2") -> ("digial output"=w205:bool)  [unwired: 7 in]
    n85 = call "Digital Pattern Generation.vi"("load data"=w198, "settings.<user name>"="settings.Pattern DIO 3", "register bus"=w193, "input.<user name>"="input.Pattern DIO 3") -> ("digial output"=w206:bool)  [unwired: 7 in]
    n86 = xnode "FPGA I/O Node"("Connector0/DIO0"=w196, "Connector0/DIO1"=w195, "Connector0/DIO2"=w205, "Connector0/DIO3"=w206) -> ()  [unwired: 4 in, 4 out]
    n87 = Unbundle By Name(w193) -> ("Crank Angle"=w192:refnum<k21>, "Cycle Angle"=w191:refnum<k21>)
    n88 = xnode ("Register Read")("Register In"=w192) -> ("Data"=w189:u16)  [unwired: 1 out]
    n89 = xnode ("Register Read")("Register In"=w191) -> ("Data"=w188:u16)  [unwired: 1 out]
    n90 = Bundle By Name(cluster=T5 {"crank"=0, "cam"=0, "crank pattern value"=FALSE, "cam pattern value"=FALSE}, "crank pattern value"=w196, "cam pattern value"=w195, "crank"=w189, "cam"=w188) -> (→"Digital Pattern Test.apu 1":T5)
  }
  n91 = node-c288(w9) -> ()
  n92 = node-c288(w39) -> ()
  n93 = node-c288() -> (w24:T23)  [unwired: 1 in]
  n94 = node-c288() -> (w22:T23)  [unwired: 1 in]
  n95 = timed-loop {
    timing: w24 -> [_]
    timing-out: [_] -> w23
    tunnel: w1 -> [w243]
    stop <- _ stop-if-true
    # "See VI context help for a description of controls and indicators"
    n96 = xnode "FPGA I/O Node"() -> ("Connector0/DIO4"=w224:bool, "Connector0/DIO5"=w223:bool, "Connector0/DIO6"=w222:bool, "Connector0/DIO7"=w221:bool, "Connector0/DIO8"=w220:bool, "Connector0/DIO9"=w219:bool)  [unwired: 6 in, 6 out]
    n97 = call-poly "Measure Events.vi"("settings.<user name>"="settings.Event DIO 4", "register bus"=w243, "event"=w224) -> ("measured data"=w242:T31, "status.<user name>"=→"status.Event DIO 4":T15)  [unwired: 7 in]
    n98 = call-poly "Measure Events.vi"("settings.<user name>"="settings.Event DIO 5", "register bus"=w243, "event"=w223) -> ("measured data"=w235:T31, "status.<user name>"=→"status.Event DIO 5":T15)  [unwired: 7 in]
    n99 = call-poly "Measure Events.vi"("settings.<user name>"="settings.Event DIO 6", "register bus"=w243, "event"=w222) -> ("measured data"=w234:T31, "status.<user name>"=→"status.Event DIO 6":T15)  [unwired: 7 in]
    n100 = call-poly "Measure Events.vi"("settings.<user name>"="settings.Event DIO 7", "register bus"=w243, "event"=w221) -> ("measured data"=w233:T31, "status.<user name>"=→"status.Event DIO 7":T15)  [unwired: 7 in]
    n101 = call-poly "Measure Events.vi"("settings.<user name>"="settings.Event DIO 8", "register bus"=w243, "event"=w220) -> ("measured data"=w232:T31, "status.<user name>"=→"status.Event DIO 8":T15)  [unwired: 7 in]
    n102 = call-poly "Measure Events.vi"("settings.<user name>"="settings.Event DIO 9", "register bus"=w243, "event"=w219) -> ("measured data"=w231:T31, "status.<user name>"=→"status.Event DIO 9":T15)  [unwired: 7 in]
    n103 = call "Capture Event.vi"("event # to capture"=T30 1 ("Settings.spark 1 shot 1"), "measured data"=w242) -> ("capture.<user name>"=→"capture.Event DIO 4.Event 1":T13)  [unwired: 9 in]
    n104 = call "Capture Event.vi"("event # to capture"=T30 1 ("Settings.spark 2 shot 1"), "measured data"=w235) -> ("capture.<user name>"=→"capture.Event DIO 5.Event 1":T13)  [unwired: 9 in]
    n105 = call "Capture Event.vi"("event # to capture"=T30 1 ("Settings.spark 3 shot 1"), "measured data"=w234) -> ("capture.<user name>"=→"capture.Event DIO 6.Event 1":T13)  [unwired: 9 in]
    n106 = call "Capture Event.vi"("event # to capture"=T30 1 ("Settings.spark 4 shot 1"), "measured data"=w233) -> ("capture.<user name>"=→"capture.Event DIO 7.Event 1":T13)  [unwired: 9 in]
    n107 = call "Capture Event.vi"("event # to capture"=T30 1 ("Settings.spark 5 shot 1"), "measured data"=w232) -> ("capture.<user name>"=→"capture.Event DIO 8.Event 1":T13)  [unwired: 9 in]
    n108 = call "Capture Event.vi"("event # to capture"=T30 1 ("Settings.spark 6 shot 1"), "measured data"=w231) -> ("capture.<user name>"=→"capture.Event DIO 9.Event 1":T13)  [unwired: 9 in]
  }
  n109 = timed-loop {
    timing: w22 -> [_]
    timing-out: [_] -> w21
    tunnel: w1 -> [w318]
    stop <- _ stop-if-true
    # "See VI context help for a description of controls and indicators"
    n110 = xnode "FPGA I/O Node"() -> ("Connector0/DIO10"=w305:bool, "Connector0/DIO11"=w304:bool, "Connector0/DIO12"=w303:bool, "Connector0/DIO13"=w302:bool, "Connector0/DIO14"=w301:bool, "Connector0/DIO15"=w300:bool)  [unwired: 6 in, 6 out]
    n111 = call-poly "Measure Events.vi"("settings.<user name>"="settings.Multi Event DIO 10", "register bus"=w318, "event"=w305) -> ("measured data"=w287:T31, "status.<user name>"=→"status.Multi Event DIO 10":T15)  [unwired: 7 in]
    n112 = call-poly "Measure Events.vi"("settings.<user name>"="settings.Multi Event DIO 11", "register bus"=w318, "event"=w304) -> ("measured data"=w280:T31, "status.<user name>"=→"status.Multi Event DIO 11":T15)  [unwired: 7 in]
    n113 = call-poly "Measure Events.vi"("settings.<user name>"="settings.Multi Event DIO 12", "register bus"=w318, "event"=w303) -> ("measured data"=w273:T31, "status.<user name>"=→"status.Multi Event DIO 12":T15)  [unwired: 7 in]
    n114 = call-poly "Measure Events.vi"("settings.<user name>"="settings.Multi Event DIO 13", "register bus"=w318, "event"=w302) -> ("measured data"=w266:T31, "status.<user name>"=→"status.Multi Event DIO 13":T15)  [unwired: 7 in]
    n115 = call-poly "Measure Events.vi"("settings.<user name>"="settings.Multi Event DIO 14", "register bus"=w318, "event"=w301) -> ("measured data"=w259:T31, "status.<user name>"=→"status.Multi Event DIO 14":T15)  [unwired: 7 in]
    n116 = call-poly "Measure Events.vi"("settings.<user name>"="settings.Multi Event DIO 15", "register bus"=w318, "event"=w300) -> ("measured data"=w252:T31, "status.<user name>"=→"status.Multi Event DIO 15":T15)  [unwired: 7 in]
    n117 = call "Capture Event.vi"("event # to capture"=T30 1 ("Settings.spark 1 shot 1"), "measured data"=w287) -> ("capture.<user name>"=→"capture.Multi Event DIO 10.Event 1":T13)  [unwired: 9 in]
    n118 = call "Capture Event.vi"("event # to capture"=T30 2 ("Settings.spark 1 shot 1"), "measured data"=w287) -> ("capture.<user name>"=→"capture.Multi Event DIO 10.Event 2":T13)  [unwired: 9 in]
    n119 = call "Capture Event.vi"("event # to capture"=T30 3 ("Settings.spark 1 shot 1"), "measured data"=w287) -> ("capture.<user name>"=→"capture.Multi Event DIO 10.Event 3":T13)  [unwired: 9 in]
    n120 = call "Capture Event.vi"("event # to capture"=T30 4 ("Settings.spark 1 shot 1"), "measured data"=w287) -> ("capture.<user name>"=→"capture.Multi Event DIO 10.Event 4":T13)  [unwired: 9 in]
    n121 = call "Capture Event.vi"("event # to capture"=T30 1 ("Settings.spark 2 shot 1"), "measured data"=w280) -> ("capture.<user name>"=→"capture.Multi Event DIO 11.Event 1":T13)  [unwired: 9 in]
    n122 = call "Capture Event.vi"("event # to capture"=T30 2 ("Settings.spark 2 shot 1"), "measured data"=w280) -> ("capture.<user name>"=→"capture.Multi Event DIO 11.Event 2":T13)  [unwired: 9 in]
    n123 = call "Capture Event.vi"("event # to capture"=T30 3 ("Settings.spark 2 shot 1"), "measured data"=w280) -> ("capture.<user name>"=→"capture.Multi Event DIO 11.Event 3":T13)  [unwired: 9 in]
    n124 = call "Capture Event.vi"("event # to capture"=T30 4 ("Settings.spark 2 shot 1"), "measured data"=w280) -> ("capture.<user name>"=→"capture.Multi Event DIO 11.Event 4":T13)  [unwired: 9 in]
    n125 = call "Capture Event.vi"("event # to capture"=T30 1 ("Settings.spark 3 shot 1"), "measured data"=w273) -> ("capture.<user name>"=→"capture.Multi Event DIO 12.Event 1":T13)  [unwired: 9 in]
    n126 = call "Capture Event.vi"("event # to capture"=T30 2 ("Settings.spark 3 shot 1"), "measured data"=w273) -> ("capture.<user name>"=→"capture.Multi Event DIO 12.Event 2":T13)  [unwired: 9 in]
    n127 = call "Capture Event.vi"("event # to capture"=T30 3 ("Settings.spark 3 shot 1"), "measured data"=w273) -> ("capture.<user name>"=→"capture.Multi Event DIO 12.Event 3":T13)  [unwired: 9 in]
    n128 = call "Capture Event.vi"("event # to capture"=T30 4 ("Settings.spark 3 shot 1"), "measured data"=w273) -> ("capture.<user name>"=→"capture.Multi Event DIO 12.Event 4":T13)  [unwired: 9 in]
    n129 = call "Capture Event.vi"("event # to capture"=T30 1 ("Settings.spark 4 shot 1"), "measured data"=w266) -> ("capture.<user name>"=→"capture.Multi Event DIO 13.Event 1":T13)  [unwired: 9 in]
    n130 = call "Capture Event.vi"("event # to capture"=T30 2 ("Settings.spark 4 shot 1"), "measured data"=w266) -> ("capture.<user name>"=→"capture.Multi Event DIO 13.Event 2":T13)  [unwired: 9 in]
    n131 = call "Capture Event.vi"("event # to capture"=T30 3 ("Settings.spark 4 shot 1"), "measured data"=w266) -> ("capture.<user name>"=→"capture.Multi Event DIO 13.Event 3":T13)  [unwired: 9 in]
    n132 = call "Capture Event.vi"("event # to capture"=T30 4 ("Settings.spark 4 shot 1"), "measured data"=w266) -> ("capture.<user name>"=→"capture.Multi Event DIO 13.Event 4":T13)  [unwired: 9 in]
    n133 = call "Capture Event.vi"("event # to capture"=T30 1 ("Settings.spark 5 shot 1"), "measured data"=w259) -> ("capture.<user name>"=→"capture.Multi Event DIO 14.Event 1":T13)  [unwired: 9 in]
    n134 = call "Capture Event.vi"("event # to capture"=T30 2 ("Settings.spark 5 shot 1"), "measured data"=w259) -> ("capture.<user name>"=→"capture.Multi Event DIO 14.Event 2":T13)  [unwired: 9 in]
    n135 = call "Capture Event.vi"("event # to capture"=T30 3 ("Settings.spark 5 shot 1"), "measured data"=w259) -> ("capture.<user name>"=→"capture.Multi Event DIO 14.Event 3":T13)  [unwired: 9 in]
    n136 = call "Capture Event.vi"("event # to capture"=T30 4 ("Settings.spark 5 shot 1"), "measured data"=w259) -> ("capture.<user name>"=→"capture.Multi Event DIO 14.Event 4":T13)  [unwired: 9 in]
    n137 = call "Capture Event.vi"("event # to capture"=T30 1 ("Settings.spark 6 shot 1"), "measured data"=w252) -> ("capture.<user name>"=→"capture.Multi Event DIO 15.Event 1":T13)  [unwired: 9 in]
    n138 = call "Capture Event.vi"("event # to capture"=T30 2 ("Settings.spark 6 shot 1"), "measured data"=w252) -> ("capture.<user name>"=→"capture.Multi Event DIO 15.Event 2":T13)  [unwired: 9 in]
    n139 = call "Capture Event.vi"("event # to capture"=T30 3 ("Settings.spark 6 shot 1"), "measured data"=w252) -> ("capture.<user name>"=→"capture.Multi Event DIO 15.Event 3":T13)  [unwired: 9 in]
    n140 = call "Capture Event.vi"("event # to capture"=T30 4 ("Settings.spark 6 shot 1"), "measured data"=w252) -> ("capture.<user name>"=→"capture.Multi Event DIO 15.Event 4":T13)  [unwired: 9 in]
  }
  n141 = node-c288(w23) -> ()
  n142 = node-c288(w21) -> ()
